vi "GT Auto Set Watch.vi"(8 "error in (no error)":errorcluster caption="错误输入（无错误）", 9 "interval":i16, 10 "pWatchInfo":i32, 11 "cardNum":i16) -> (0 "error out":errorcluster caption="错误输出", 2 "pWatchInfo out":i32, 3 "cardNum":i16)   [LabVIEW 2020, in "gts1.lvlib"]
doc: "GT_API GT_AutoSetWatch(short cardNum,long *pWatchInfo,short interval);"
uses:
  gts1.lvlib
  dll/32bit/multi_card/gts.dll
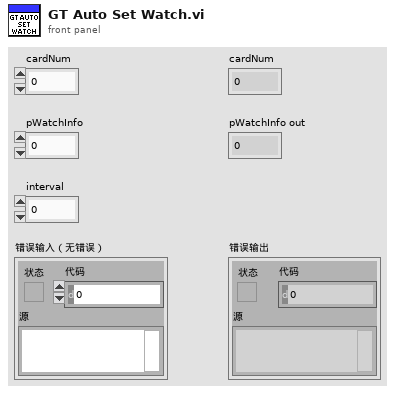
[diagram p1: front panel]
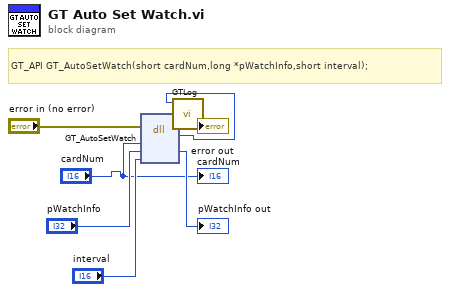
[diagram p0: block diagram]
diagram:
  # "GT_API GT_AutoSetWatch(short cardNum,long *pWatchInfo,short interval);"
  n1 = dll-call lib="D:/Git/GoogolCard/dll/32bit/multi_card/gts.dll" fn="GT_AutoSetWatch"(error in="error in (no error)", "cardNum"="cardNum", "pWatchInfo"="pWatchInfo", "interval"="interval") -> (error out=w4:errorcluster, w2:i16, "pWatchInfo"=→"pWatchInfo out":i32)  [unwired: 4 in, 1 out]
  n2 = call "GTLog.vi"("error in (no error)"=w4, "Numeric"=w2) -> ("error out"=→"error out":errorcluster)  [unwired: 9 in]
  "cardNum" <- "cardNum"
